vi "Auton - Center Gear Shoot.vi"(9 "Alliance":T2, 11 "Auton States":T1=enum."Reset Encoders") -> ()   [LabVIEW 2016]
uses:
  Auton - Center Gear Shoot States.ctl
  <vilib>/Rock Robotics/WPI/DriverStation/WPI_DriverStationAllianceInfo.ctl
  Robot Values.vi
panel:
  in  "Drive Toward Boiler":dbl=100.0
  in  "Blue - Turn toward Boiler":dbl=270.0 format="%#_13g"
  in  "Red - Turn Toward Boiler SP":dbl=90.0 format="%#_13g"
  in  "Back Away Gear SP":dbl=-36.0
  out "Auton States":T1=enum."Reset Encoders"
  in  "High Speed Output Range":cluster{"output high":dbl, "output low":dbl}={"output high"=0.9, "output low"=-0.9}
  in  "Blue - Turn to Boiler":dbl=215.0 format="%#_13g"
  in  "Red - Turn to Boiler SP":dbl=135.0 format="%#_13g"
  in  "Move to Boiler SP":dbl=22.0
  in  "Red - Mount Angle Setpoint":dbl=9.0 format="%#_13g"
  in  "Mount Gear":dbl=9.0
  in  "Blue - Mount Angle Setpoint":dbl=9.0 format="%#_13g"
  in  "Drive Forward SP":dbl=60.0
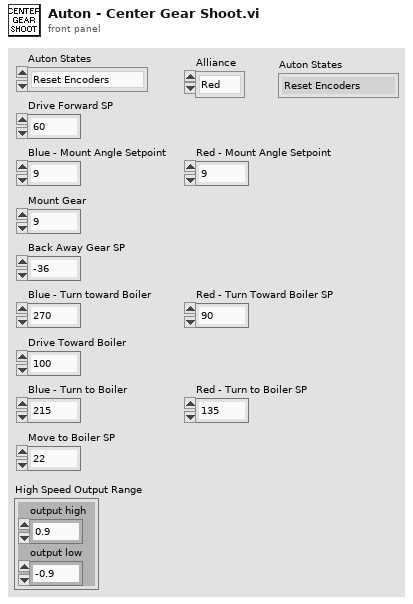
[diagram p1: front panel]
types:
  T1 = typedef "Auton - Center Gear Shoot States.ctl" = enum16{"Stop", "Reset Encoders", "Go to Target", "Turn to Mount Gear", "Reset Encoders Mount", "Mount Gear", "Eject Gear", "Back Away from Gear", "Turn Toward Boiler", "Reset Encoder Toward Boiler", "Drive Toward Boiler", "Turn to Boiler", "Reset Encoders Boiler", "Move to Boiler", "Shoot"}
  T2 = typedef "WPI_DriverStationAllianceInfo.ctl" = enum16{"Red", "Blue", "Invalid"}
  T3 = typedef "Robot Values.ctl" = cluster{"Robot Drive":cluster{"Left Motor Power":dbl, "Right Motor Power":dbl, "Left Encoder Value":dbl, "Right Encoder Value":dbl, "High Gear?":bool, "PTO?":bool}, "Sensors":cluster{"Gyro Angle":u16, "Recalibrate Gyro":bool, "Reset Gyro":bool, "Ultrasonic":dbl}, "Shooter":cluster{"Prep Wheels":bool, "Shoot":bool, "Left Shooter Wheel Speed":dbl, "Wheels Moving":bool, "Shooter Prepped":bool, "Shooter RPS SP":dbl, "Shooting?":bool, "Left Shooter Wheel Power":dbl, "Right Shooter Wheel Power":dbl, "Acquisition Conveyor Power":dbl, "Hopper Beater Bar Power":dbl, "Filtered Left Shooter Speed":dbl, "Acquisition Motor Power":dbl, "Joystick Add":dbl}, "Robot States":cluster{"Drive mode":string, "Alliance":T2, "Position":T4}, "Gear":cluster{"Ejection Active":bool}}
  T4 = typedef "WPI_DriverStationPositionInfo.ctl" = enum16{"1", "2", "3"}
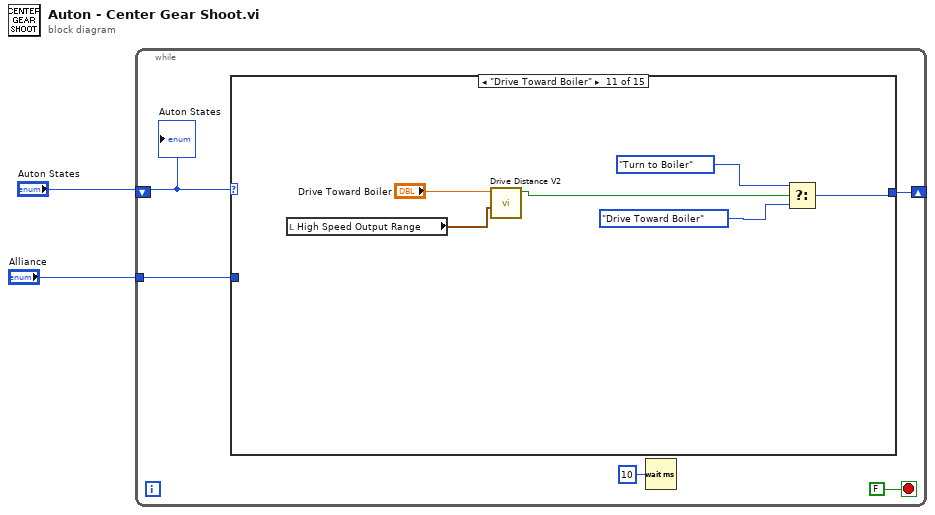
[diagram p0: block diagram]
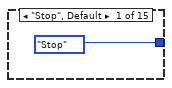
[diagram p2: hidden frame]
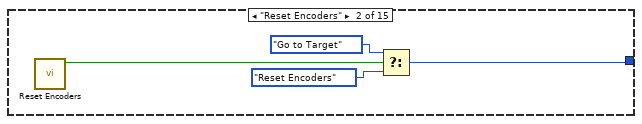
[diagram p3: hidden frame]
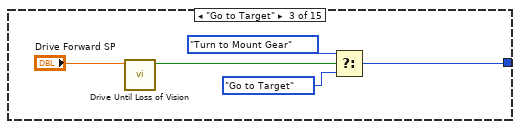
[diagram p4: hidden frame]
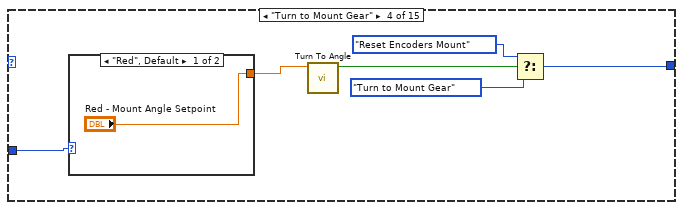
[diagram p5: hidden frame]
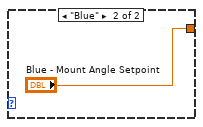
[diagram p6: hidden frame]
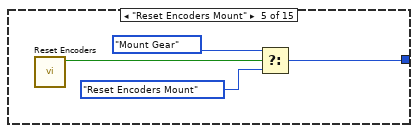
[diagram p7: hidden frame]
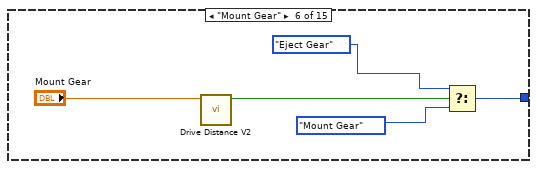
[diagram p8: hidden frame]
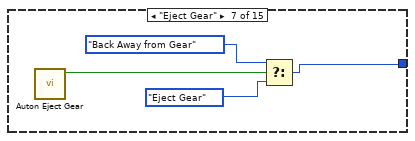
[diagram p9: hidden frame]
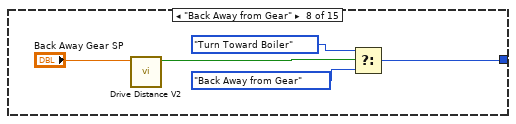
[diagram p10: hidden frame]
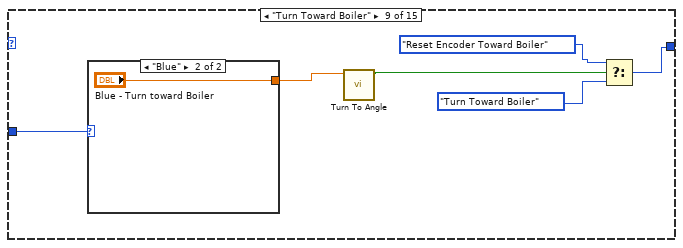
[diagram p11: hidden frame]
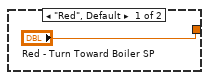
[diagram p12: hidden frame]
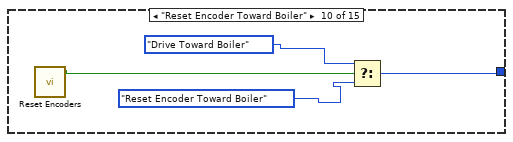
[diagram p13: hidden frame]
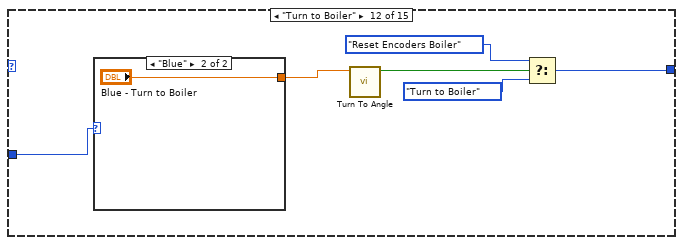
[diagram p14: hidden frame]
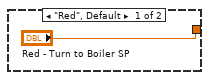
[diagram p15: hidden frame]
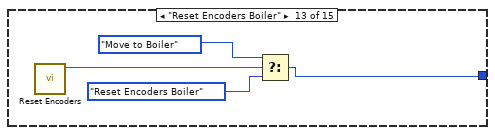
[diagram p16: hidden frame]
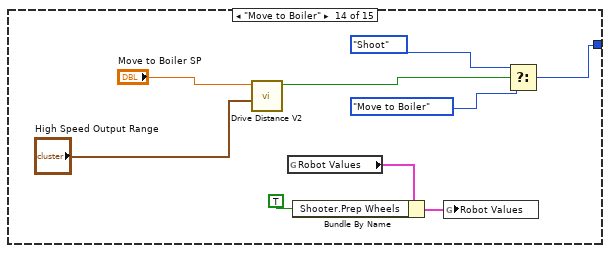
[diagram p17: hidden frame]
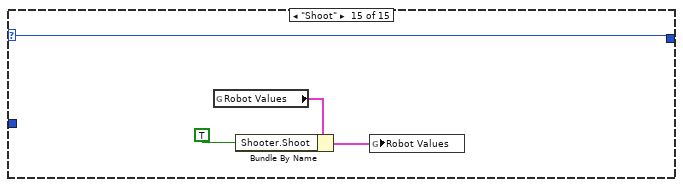
[diagram p18: hidden frame]
diagram:
  n1 = while {
    shift-right: [w6] -> _
    shift-left: "Auton States" -> [w7]
    tunnel: "Alliance" -> [w5]
    stop <- FALSE stop-if-true
    n2 = case shown="\"Drive Toward Boiler\"" w7 {
      selector: w7 -> [_ _ _ _ _ _ _ _ _ _ _ _ _ _ w83]
      tunnel: [Auton_-_Center_Gear_Shoot_States."Stop" ("Auton States") w11 w17 w23 w29 w34 w38 w43 w49 w55 w61 w65 w72 w80 w83] -> w6
      tunnel: w5 -> [_ _ _ w20 _ _ _ _ w45 _ _ w64 _ _ _]
      frame "Stop", Default {
      }
      frame "Reset Encoders" {
        n3 = call "Reset Encoders.vi"() -> ("Done?"=w12:bool)  [unwired: 11 in]
        n4 = Select(t=Auton_-_Center_Gear_Shoot_States."Go to Target" ("Auton States"), s=w12, f=Auton_-_Center_Gear_Shoot_States."Reset Encoders" ("Auton States")) -> (s? t:f=w11:T1)
      }
      frame "Go to Target" {
        n5 = call "Drive Until Loss of Vision.vi"("Distance Setpoint"="Drive Forward SP") -> ("ready to approach"=w13:bool)  [unwired: 10 in]
        n6 = Select(t=Auton_-_Center_Gear_Shoot_States."Turn to Mount Gear" ("Auton States"), s=w13, f=Auton_-_Center_Gear_Shoot_States."Go to Target" ("Auton States")) -> (s? t:f=w17:T1)
      }
      frame "Turn to Mount Gear" {
        n7 = case shown="\"Red\", Default" w20 {
          tunnel: ["Red - Mount Angle Setpoint" "Blue - Mount Angle Setpoint"] -> w21
          frame "Red", Default {
          }
          frame "Blue" {
          }
        }
        n8 = call "Turn To Angle.vi"("Setpoint"=w21) -> ("Done?"=w22:bool)  [unwired: 10 in]
        n9 = Select(t=Auton_-_Center_Gear_Shoot_States."Reset Encoders Mount" ("Auton States"), s=w22, f=Auton_-_Center_Gear_Shoot_States."Turn to Mount Gear" ("Auton States")) -> (s? t:f=w23:T1)
      }
      frame "Reset Encoders Mount" {
        n10 = call "Reset Encoders.vi"() -> ("Done?"=w28:bool)  [unwired: 11 in]
        n11 = Select(t=Auton_-_Center_Gear_Shoot_States."Mount Gear" ("Auton States"), s=w28, f=Auton_-_Center_Gear_Shoot_States."Reset Encoders Mount" ("Auton States")) -> (s? t:f=w29:T1)
      }
      frame "Mount Gear" {
        n12 = call "Drive Distance V2.vi"("Distance Set Point"="Mount Gear") -> ("Done?"=w33:bool)  [unwired: 10 in]
        n13 = Select(t=Auton_-_Center_Gear_Shoot_States."Eject Gear" ("Auton States"), s=w33, f=Auton_-_Center_Gear_Shoot_States."Mount Gear" ("Auton States")) -> (s? t:f=w34:T1)
      }
      frame "Eject Gear" {
        n14 = call "Auton Eject Gear.vi"() -> ("Done?"=w35:bool)  [unwired: 11 in]
        n15 = Select(t=Auton_-_Center_Gear_Shoot_States."Back Away from Gear" ("Auton States"), s=w35, f=Auton_-_Center_Gear_Shoot_States."Eject Gear" ("Auton States")) -> (s? t:f=w38:T1)
      }
      frame "Back Away from Gear" {
        n16 = call "Drive Distance V2.vi"("Distance Set Point"="Back Away Gear SP") -> ("Done?"=w39:bool)  [unwired: 10 in]
        n17 = Select(t=Auton_-_Center_Gear_Shoot_States."Turn Toward Boiler" ("Auton States"), s=w39, f=Auton_-_Center_Gear_Shoot_States."Back Away from Gear" ("Auton States")) -> (s? t:f=w43:T1)
      }
      frame "Turn Toward Boiler" {
        n18 = case shown="\"Blue\"" w45 {
          tunnel: ["Red - Turn Toward Boiler SP" "Blue - Turn toward Boiler"] -> w46
          frame "Red", Default {
          }
          frame "Blue" {
          }
        }
        n19 = call "Turn To Angle.vi"("Setpoint"=w46) -> ("Done?"=w44:bool)  [unwired: 10 in]
        n20 = Select(t=Auton_-_Center_Gear_Shoot_States."Reset Encoder Toward Boiler" ("Auton States"), s=w44, f=Auton_-_Center_Gear_Shoot_States."Turn Toward Boiler" ("Auton States")) -> (s? t:f=w49:T1)
      }
      frame "Reset Encoder Toward Boiler" {
        n21 = call "Reset Encoders.vi"() -> ("Done?"=w52:bool)  [unwired: 11 in]
        n22 = Select(t=Auton_-_Center_Gear_Shoot_States."Drive Toward Boiler" ("Auton States"), s=w52, f=Auton_-_Center_Gear_Shoot_States."Reset Encoder Toward Boiler" ("Auton States")) -> (s? t:f=w55:T1)
      }
      frame "Drive Toward Boiler" {
        n23 = local read "High Speed Output Range"() -> (w56:cluster{"output high":dbl, "output low":dbl})
        n24 = call "Drive Distance V2.vi"("output range"=w56, "Distance Set Point"="Drive Toward Boiler") -> ("Done?"=w57:bool)  [unwired: 9 in]
        n25 = Select(t=Auton_-_Center_Gear_Shoot_States."Turn to Boiler" ("Auton States"), s=w57, f=Auton_-_Center_Gear_Shoot_States."Drive Toward Boiler" ("Auton States")) -> (s? t:f=w61:T1)
      }
      frame "Turn to Boiler" {
        n26 = case shown="\"Blue\"" w64 {
          tunnel: ["Red - Turn to Boiler SP" "Blue - Turn to Boiler"] -> w66
          frame "Red", Default {
          }
          frame "Blue" {
          }
        }
        n27 = call "Turn To Angle.vi"("Setpoint"=w66) -> ("Done?"=w67:bool)  [unwired: 10 in]
        n28 = Select(t=Auton_-_Center_Gear_Shoot_States."Reset Encoders Boiler" ("Auton States"), s=w67, f=Auton_-_Center_Gear_Shoot_States."Turn to Boiler" ("Auton States")) -> (s? t:f=w65:T1)
      }
      frame "Reset Encoders Boiler" {
        n29 = call "Reset Encoders.vi"() -> ("Done?"=w73:bool)  [unwired: 11 in]
        n30 = Select(t=Auton_-_Center_Gear_Shoot_States."Move to Boiler" ("Auton States"), s=w73, f=Auton_-_Center_Gear_Shoot_States."Reset Encoders Boiler" ("Auton States")) -> (s? t:f=w72:T1)
      }
      frame "Move to Boiler" {
        n31 = call "Drive Distance V2.vi"("output range"="High Speed Output Range", "Distance Set Point"="Move to Boiler SP") -> ("Done?"=w81:bool)  [unwired: 9 in]
        n32 = global read "Robot Values.vi" "Robot Values"() -> (w79:T3)
        n33 = Bundle By Name(cluster=w79, "Shooter.Prep Wheels"=TRUE) -> (w78:T3)
        n34 = global write "Robot Values.vi" "Robot Values"(w78) -> ()
        n35 = Select(t=Auton_-_Center_Gear_Shoot_States."Shoot" ("Auton States"), s=w81, f=Auton_-_Center_Gear_Shoot_States."Move to Boiler" ("Auton States")) -> (s? t:f=w80:T1)
      }
      frame "Shoot" {
        n36 = global read "Robot Values.vi" "Robot Values"() -> (w86:T3)
        n37 = Bundle By Name(cluster=w86, "Shooter.Shoot"=TRUE ("Shooter.Prep Wheels")) -> (w85:T3)
        n38 = global write "Robot Values.vi" "Robot Values"(w85) -> ()
      }
    }
    n39 = Wait (ms)(milliseconds to wait=u32 10) -> ()  [unwired: 1 out]
    "Auton States" <- w7
  }
